vi "Emergency_Stop.vi"() -> ()   [LabVIEW 2010]
panel:
  in  "stop":bool
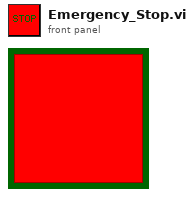
[diagram p1: front panel]
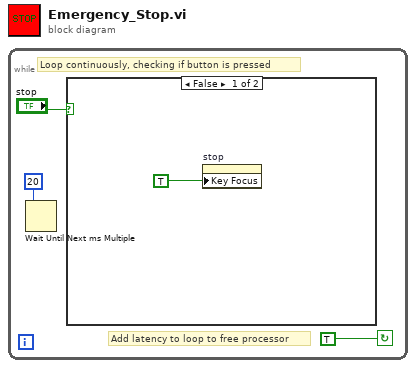
[diagram p0: block diagram]
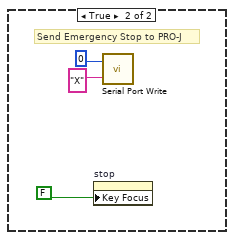
[diagram p2: hidden frame]
diagram:
  n1 = while {
    stop <- TRUE continue-if-true
    # "Add latency to loop to free processor"
    # "Loop continuously, checking if button is pressed"
    n2 = Wait Until Next ms Multiple(millisecond multiple=20) -> ()  [unwired: 1 out]
    n3 = case shown="False" "stop" {
      frame False {
        n4 = property on="stop" class="Bool"("Key Focus"=TRUE) -> ()  [unwired: 2 in, 2 out]
      }
      frame True {
        # "Send Emergency Stop to PRO-J"
        n5 = property on="stop" class="Bool"("Key Focus"=FALSE) -> ()  [unwired: 2 in, 2 out]
        n6 = call <vilib>:"Serial Port Write.vi"("string to write"="X", "port number"=0) -> ()  [unwired: 1 out]
      }
    }
  }
